vi "pendant_OC basic.vi"() -> ()   [LabVIEW 2014]
uses:
  <vilib>/Utility/miscctls.llb/LVBoundsTypeDef.ctl
  <vilib>/DAQmx/create/channels.llb/DAQmx Create Channel (AI-Voltage-Basic).vi
  <vilib>/DAQmx/configure/timing.llb/DAQmx Timing (Sample Clock).vi
  <vilib>/ethernetip/ethernetip.lvlib
panel:
  in  "Boolean 12":bool
  out "String 17":string="RECONNECT\nTRANSDUCER"
  out "Hz":dbl format="%05.1g"
  out "Trq":dbl format="%05.1g"
  in  "OK Button":bool
  out "Network Error":string="NETWORK\nERROR"
  out "DAQ READ ERROR":string
  out "HIMMELSTEIN READ ERROR":string
  out "DRIVE READ ERROR":string
  in  "Boolean 11":bool
  out "String 15":string="60HZ LOCK"
  in  "Boolean 7":bool=TRUE
  out "String 8":string="ADJ"
  in  "speed control":dbl(slide) max=100.0 step=0.1 scale=0.0..100.0 scale format="%05.1f"
  in  "Boolean 10":bool=TRUE
  out "String 9":string="ADJ"
  in  "trq control":dbl(slide) step=0.01 scale=0.0..100.0 scale format="%06.2g"
  in  "Boolean 9":bool
  in  "Boolean 5":bool
  out "String 14":string="RECONNECT\nTRANSDUCER"
  out "Numeric 10":dbl format="%_3g"
  out "2D Picture 7":picture
  out "String 13":string="PROBE\nERROR"
  out "String 12":string="TRANSDUCER\nERROR"
  out "String 10":string="ALARM"
  in  "Boolean 6":bool
  out "String 7":string="FAULT"
  out "Numeric 9":dbl format="%4_4g"
  out "2D Picture 6":picture
  in  "REV RUN":bool
  out "String 5":string="REV RUN"
  in  "FWD RUN":bool
  out "String 3":string="FWD RUN"
  in  "Boolean 3":bool
  out "String 4":string="STOP"
  out "Numeric 8":dbl format="%4_4g"
  out "2D Picture 5":picture
  out "Numeric 7":dbl format="%4_4g"
  out "2D Picture 4":picture
  out "Amps":dbl format="%05.1f"
  out "HP":dbl format="%05.1f"
  out "LB-FT":dbl format="%06.1f"
  out "RPM":dbl format="%06.1f"
  out "% Torque":dbl format="%05.1g"
  out "Hz":dbl format="%05.1g"
  in  "Dyne in use:":string(combo)
  in  "stop":bool
  out "Load Drive:":string
  # "Load Speed Actual:"
  # "Load Torque % Actual:"
  # "Speed \nRef/Lim (Hz)"
  # "Torque \nRef/Lim (%)"
  # "Current\nOnly"
  # "Average of 3 current probes"
  # "Yaskawa America, Inc."
  # "TEST DRIVE REGEN:\nset > test drive speed"
  # "Pendant style load controller"
  # "2018"
  # "v0.1"
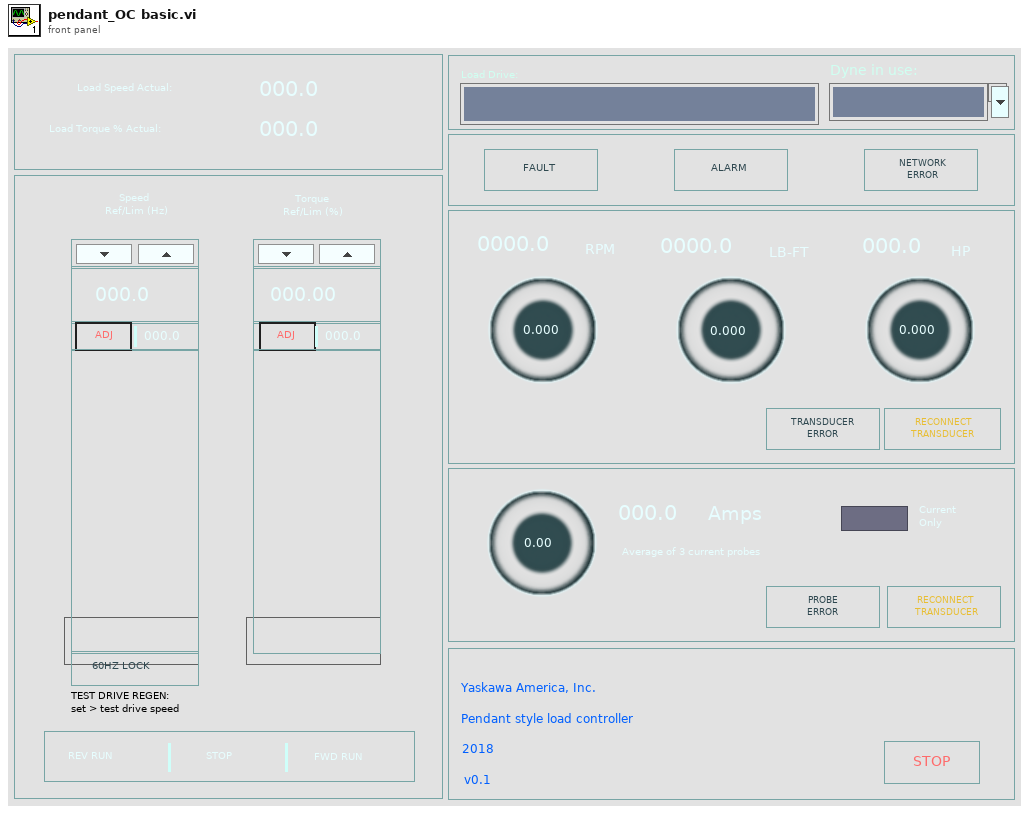
[diagram p1: front panel]
types:
  T1 = enum16{"[A1-02] Control Method Selection (general) [TEXT]", "[b1-01] Reference Source 1 (general) [TEXT]", "[b1-02] Run Source 1 (general) [TEXT]", "[b1-03] Stopping Method Selection (general) [TEXT]", "[C1-01] Acceleration Time 1 (general) [NUMERIC]", "[C1-02] Deceleration Time 1 (general) [NUMERIC]", "[C4-01] Torque Compensation Gain (general) [NUMERIC]", "[C6-01] Drive Duty Selection (general) [TEXT]", "[C6-02] Carrier Frequency Selection (general) [TEXT]", "[d1-01] Frequency Reference 1 (general) [NUMERIC]", "[H4-01] Multi-Function Analog Output Terminal FM Monitor Selection (general) [TEXT]", "[H4-02] Multi-Function Analog Output Terminal FM Gain (general) [NUMERIC]", "[H4-03] Multi-Function Analog Output Terminal FM Bias (general) [NUMERIC]", "[H4-04] Multi-Function Analog Output Terminal AM Monitor Selection (general) [TEXT]", "[H4-05] Multi-Function Analog Output Terminal AM Gain (general) [NUMERIC]", "[H4-06] Multi-Function Analog Output Terminal AM Bias (general) [NUMERIC]", "[L1-01] Motor Overload Protection Selection (general) [TEXT]", "[L3-01] Stall Prevention Selection during Acceleration (general) [TEXT]", "[L3-04] Stall Prevention Selection during Deceleration (general) [TEXT]", "[L3-05] Stall Prevention Selection during Run (general) [TEXT]", "[L8-14] Drive Overload (oL2) Protection Selection (general) [TEXT]", "[n1-01] Hunting Prevention Selection (general) [TEXT]", "[o2-04] Drive Model Selection (general) [TEXT]", "[C2-01] S-Curve Characteristic at Accel Start (S-Curve) [NUMERIC]", "[C2-02] S-Curve Characteristic at Accel End (S-Curve) [NUMERIC]", "[E1-03] V/f Pattern Selection (V/f Pattern) [TEXT]", "[E1-04] Maximum Output Frequency (V/f Pattern) [NUMERIC]", "[E1-05] Maximum Voltage (V/f Pattern) [NUMERIC]", "[E1-06] Base Frequency (V/f Pattern) [NUMERIC]", "[E1-07] Middle Output Frequency (V/f Pattern) [NUMERIC]", "[E1-08] Middle Output Frequency Voltage (V/f Pattern) [NUMERIC]", "[E1-09] Minimum Output Frequency (V/f Pattern) [NUMERIC]", "[E1-10] Minimum Output Frequency Voltage (V/f Pattern) [NUMERIC]", "[E2-01] Motor Rated Current (Motor Parameters) [NUMERIC]", "[E2-03] Motor No-Load Current (Motor Parameters) [NUMERIC]", "[E2-04] Number of Motor Poles (Motor Parameters) [NUMERIC]", "[E2-11] Motor Rated Power (Motor Parameters) [NUMERIC]", "[L1-13] Continuous Electrothermal Operation Selection (Memory Retention) [TEXT]", "[H1-01] Term S1 Func Sel (DI control) [TEXT]", "[H1-02] Term S2 Func Sel (DI control) [TEXT]", "[H1-03] Term S3 Func Sel (DI control) [TEXT]", "[H1-04] Term S4 Func Sel (DI control) [TEXT]", "[H1-05] Term S5 Func Sel (DI control) [TEXT]", "[H1-06] Term S6 Func Sel (DI control) [TEXT]", "[H1-07] Term S7 Func Sel (DI control) [TEXT]", "[H1-08] Term S8 Func Sel (DI control) [TEXT]", "[H3-01] Term A1 Level (AI control) [TEXT]", "[H3-02] Term A1 FuncSel (AI control) [TEXT]", "[H3-03] Term A1 Gain (AI control) [NUMERIC]", "[H3-04] Term A1 Bias (AI control) [NUMERIC]", "[H3-05] Term A3 Signal (AI control) [TEXT]", "[H3-06] Term A3 Sel (AI control) [TEXT]", "[H3-07] Term A3 Gain (AI control) [NUMERIC]", "[H3-08] Term A3 Bias (AI control) [NUMERIC]", "[H3-09] Term A2 Level (AI control) [TEXT]", "[H3-10] Term A2 FuncSel (AI control) [TEXT]", "[H3-11] Term A2 Gain (AI control) [NUMERIC]", "[H3-12] Term A2 Bias (AI control) [NUMERIC]"}
  T2 = enum16{"output frequency [U1-02]", "output current [U1-03]", "control method [U1-04]", "output voltage reference [U1-06]", "DC bus voltage [U1-07]", "output power [U1-08]"}
  T3 = typedef "LVBoundsTypeDef.ctl" = cluster{"Width":u32, "Height":u32}
  T4 = cluster{"Width":u32, "Width":u32, "Width":u32, "Height":u32}
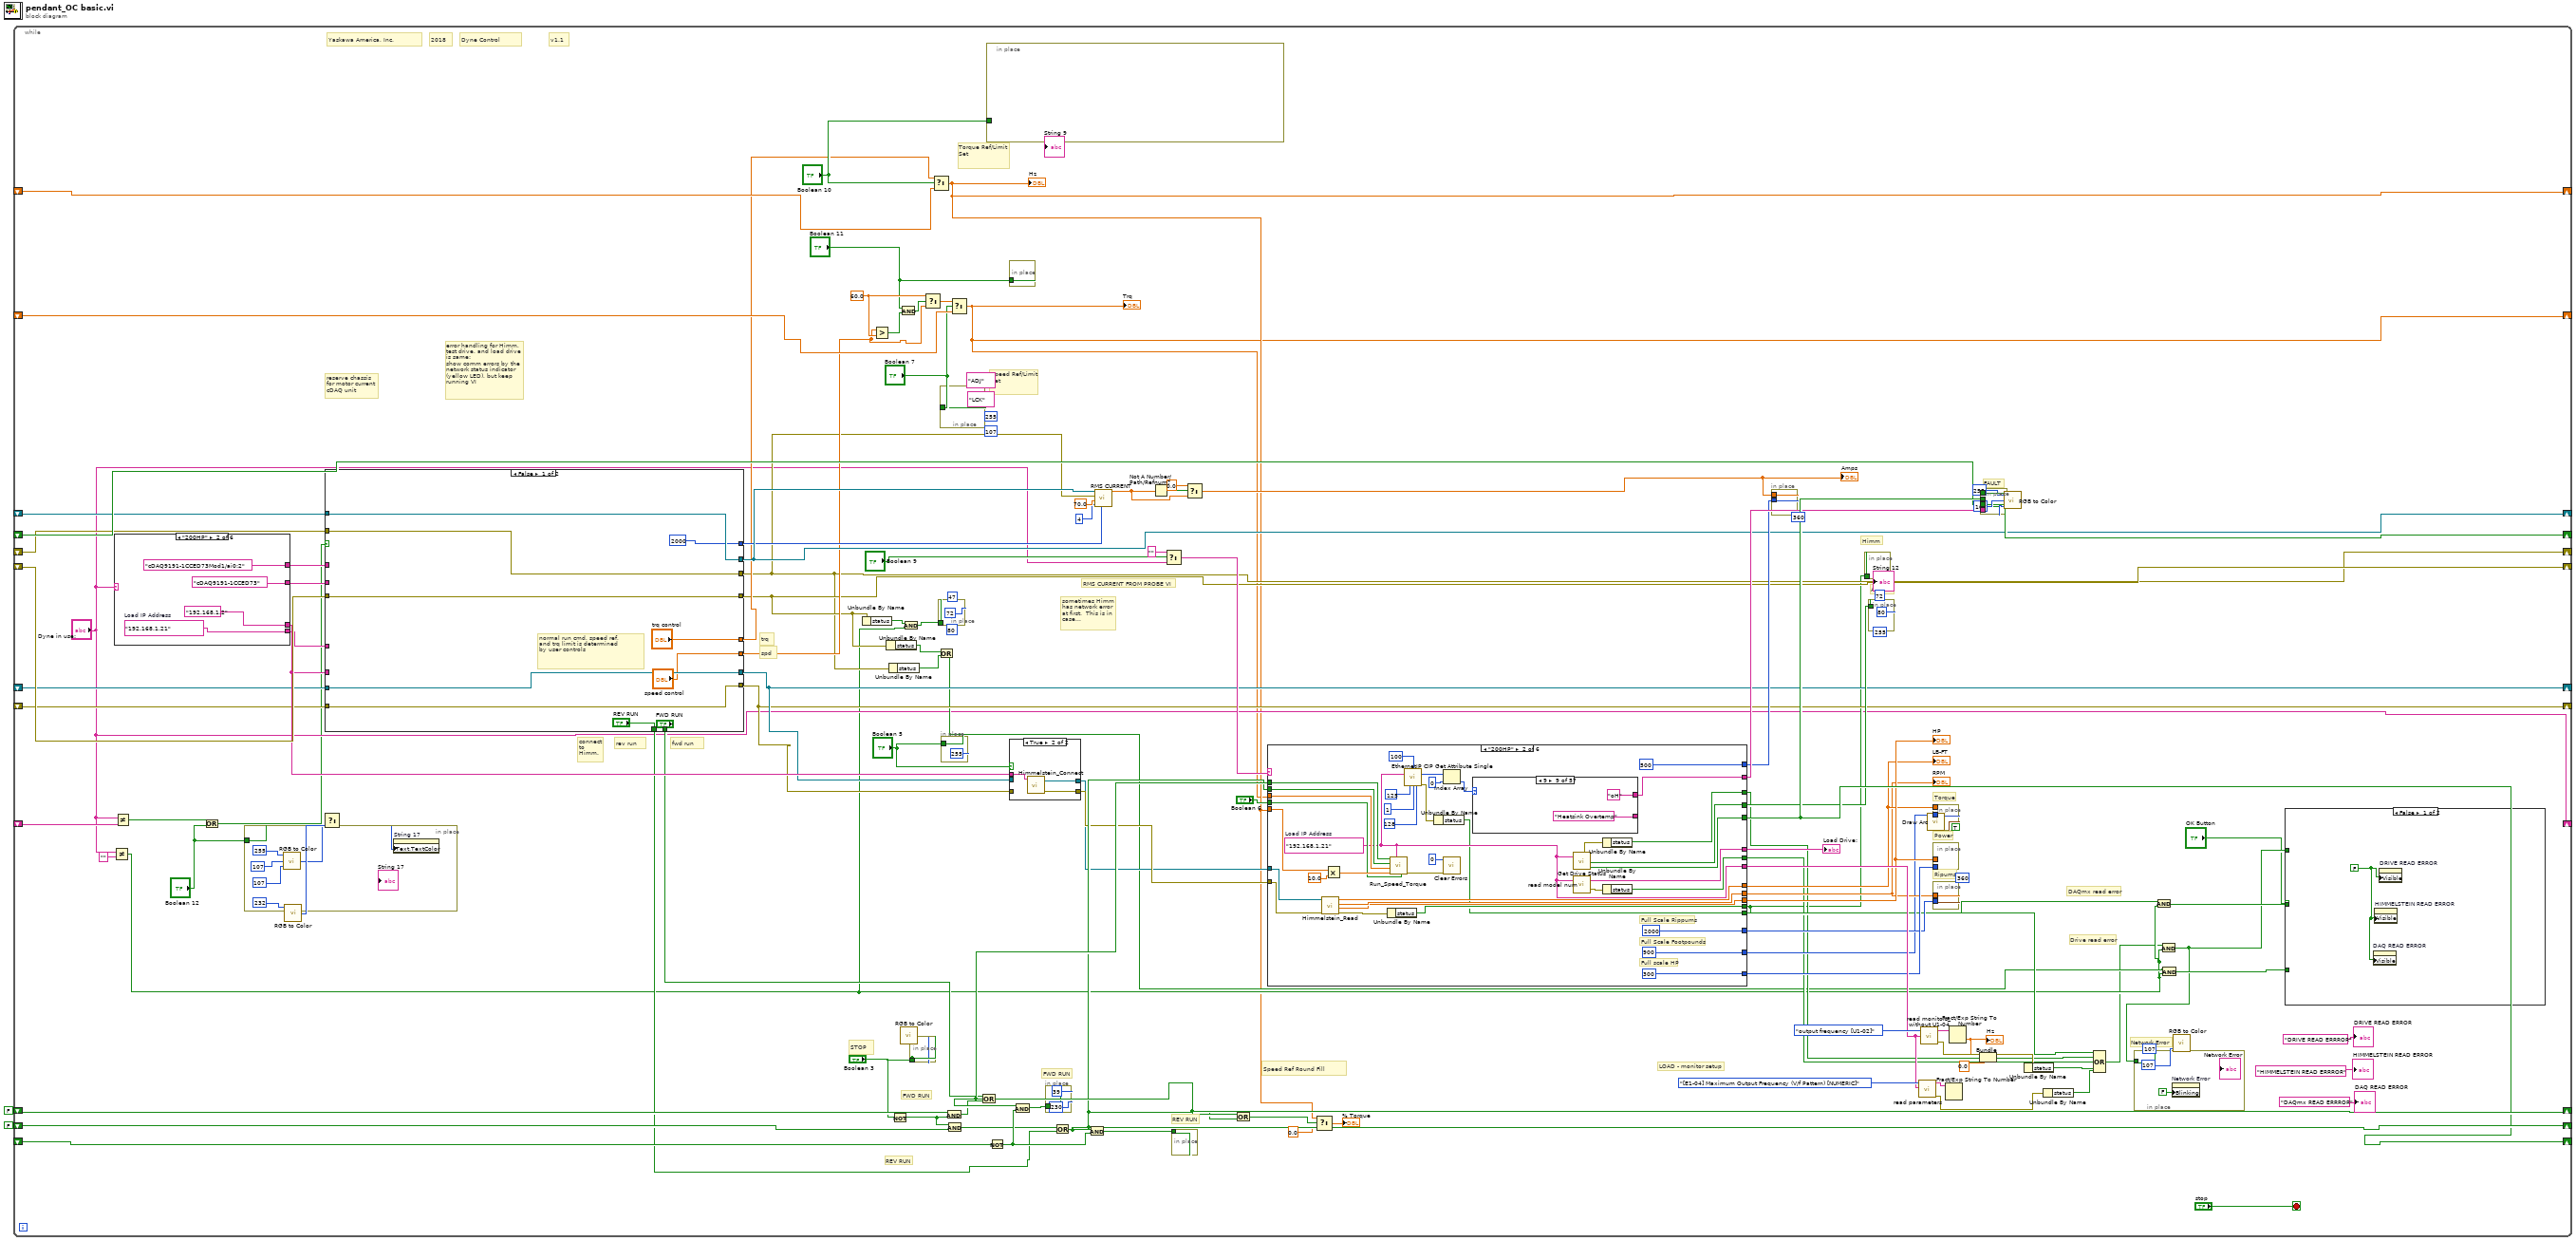
[diagram p0: block diagram]
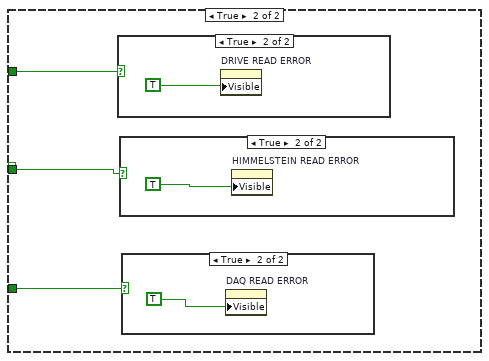
[diagram p2: hidden frame]
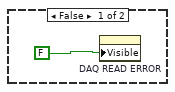
[diagram p3: hidden frame]
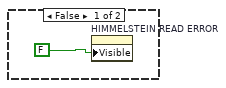
[diagram p4: hidden frame]
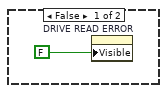
[diagram p5: hidden frame]
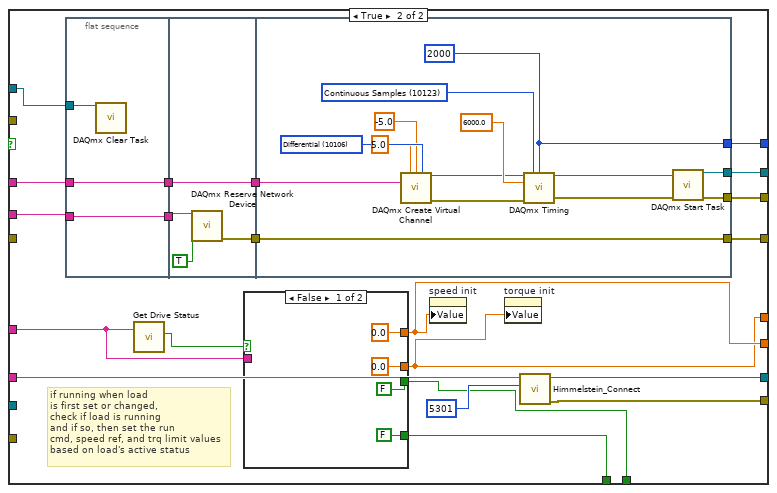
[diagram p6: hidden frame]
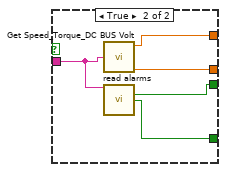
[diagram p7: hidden frame]
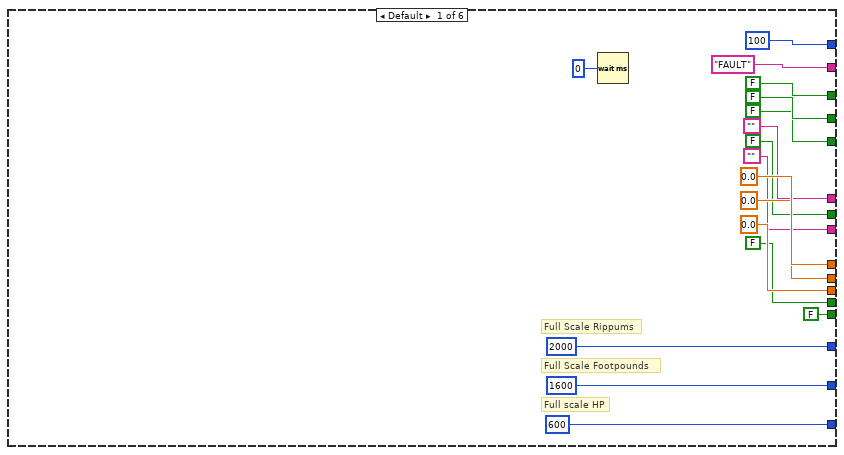
[diagram p9: hidden frame]
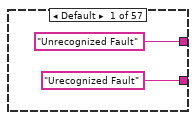
[diagram p10: hidden frame]
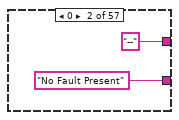
[diagram p11: hidden frame]
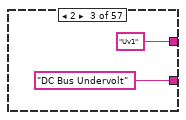
[diagram p12: hidden frame]
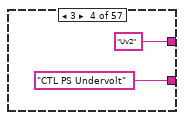
[diagram p13: hidden frame]
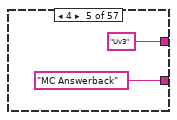
[diagram p14: hidden frame]
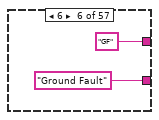
[diagram p15: hidden frame]
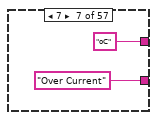
[diagram p16: hidden frame]
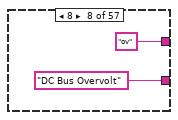
[diagram p17: hidden frame]
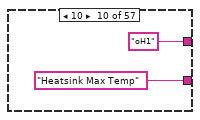
[diagram p18: hidden frame]
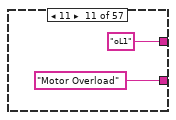
[diagram p19: hidden frame]
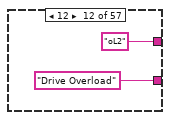
[diagram p20: hidden frame]
diagram:
  n1 = while {
    shift-right: [w107] -> _
    shift-left: FALSE -> [w104]
    shift-right: [w106] -> _
    shift-left: FALSE -> [w103]
    shift-right: [w105] -> _
    shift-left: _ -> [w102]
    shift-right: [w7] -> _
    shift-left: _ -> [w100]
    shift-right: [w6] -> _
    shift-left: _ -> [w101]
    shift-right: [w99] -> _
    shift-left: _ -> [w98]
    shift-right: ["Dyne in use:"] -> _
    shift-left: _ -> [w53]
    shift-right: [w25] -> _
    shift-left: _ -> [w50]
    shift-right: [w52] -> _
    shift-left: _ -> [w51]
    shift-right: [w26] -> _
    shift-left: _ -> [w49]
    shift-right: [w46] -> _
    shift-left: _ -> [w44]
    shift-right: [w45] -> _
    shift-left: _ -> [w43]
    stop <- "stop" stop-if-true
    w73 = 60.0 ("t")
    # "DAQmx read error"
    # "Drive read error"
    # "rev run"
    # "fwd run"
    # "spd"
    # "trq"
    # "REV RUN"
    # "FWD RUN"
    # "Network Error"
    # "ALARM"
    # "REV RUN"
    # "STOP"
    # "sometimes Himm\nhas network error \nat first.  This is in\ncase..."
    # "Speed Ref Round Fill"
    # "Speed Ref/Limit Set"
    # "Torque Ref/Limit Set"
    # "FAULT"
    # "FWD RUN"
    # "LOAD - monitor setup"
    # "Himm"
    # "RMS CURRENT FROM PROBE VI"
    # "Torque"
    # "Power"
    # "Ripums"
    # "reserve chassis \nfor motor current\ncDAQ unit"
    # "error handling for Himm,\ntest drive, and load drive\nis same:\nshow comm errors by the \nnetwork status indicator \n(yellow LED), but keep\nrunning VI"
    # "connect\nto \nHimm."
    # "Dyne Control"
    # "v1.1"
    # "2018"
    # "Yaskawa America, Inc."
    n2 = Not Equal?(x="Dyne in use:", y="") -> (x != y?=w11:bool)
    n3 = case shown="\"200HP\"" "Dyne in use:" {
      tunnel: [tag "" ("device in") tag "cDAQ9191-1CCED73" ("device in") tag "" ("device in") tag "cDAQ9191-1CCED79" ("device in") tag "cDAQ9191-1CCED73" ("device in") tag "cDAQ9191-1CCED73" ("device in")] -> w109
      tunnel: ["" "192.168.1.2" "" "192.168.1.3" "192.168.1.5" "192.168.1.4"] -> w47
      tunnel: [tag "" ("physical channels") tag "cDAQ9191-1CCED73Mod1/ai0:2" ("physical channels") tag "" ("physical channels") tag "cDAQ9191-1CCED79Mod1/ai0:2" ("physical channels") tag "cDAQ9191-1CCED73Mod1/ai0:2" ("physical channels") tag "cDAQ9191-1CCED73Mod1/ai0:2" ("physical channels")] -> w108
      tunnel: [w1160 w1164 w1168 w1172 w1176 w1180] -> w36
      frame Default {
        w1160 = ""  # Load IP Address
      }
      frame "200HP" {
        w1164 = "192.168.1.21"  # Load IP Address
      }
      frame "Portable Stand" {
        w1168 = "192.168.1.20"  # Load IP Address
      }
      frame "500HP" {
        w1172 = "192.168.1.22"  # Load IP Address
      }
      frame "1200HP" {
        w1176 = "192.168.1.23"  # Load IP Address
      }
      frame "600HP" {
        w1180 = "192.168.1.23"  # Load IP Address
      }
    }
    n4 = Not Equal?(x="Dyne in use:", y=w53) -> (x != y?=w5:bool)
    n5 = Or(x=w5, y="Boolean 12") -> (x .or. y?=w4:bool)
    n6 = in-place {
      in-place-border: "Boolean 12" -> [w113]
      # "reconnect"
      n7 = call <vilib>:"RGB to Color.vi"("B"=u8 107 ("R"), "G"=u8 107 ("R"), "R"=u8 255) -> ("Color"=w111:u32)
      n8 = call <vilib>:"RGB to Color.vi"("B"=u8 51 ("R"), "G"=u8 190 ("R"), "R"=u8 232) -> ("Color"=w112:u32)
      n9 = Select(t=w111, s=w113, f=w112) -> (s? t:f=w110:u32)
      n10 = property on="String 17" class="Str"("Text.TextColor"=w110) -> ()  [unwired: 2 in, 2 out]
    }
    n11 = case shown="False" w4 {
      tunnel: w109 -> [_ w158]
      tunnel: [w137 w157] -> w26
      tunnel: w108 -> [_ w156]
      tunnel: [w139 w155] -> w52
      tunnel: [w138 w154] -> w25
      tunnel: w51 -> [w139 w146]
      tunnel: w50 -> [w138 _]
      tunnel: w49 -> [w137 _]
      tunnel: [w136 w153] -> w46
      tunnel: [w135 w152] -> w45
      tunnel: w47 -> [_ w151]
      tunnel: w44 -> [w136 _]
      tunnel: w43 -> [w135 _]
      tunnel: [2000 ("samples per channel") w149] -> w37
      tunnel: w36 -> [_ w144]
      tunnel: ["trq control" w142] -> w35
      tunnel: ["speed control" w143] -> w34
      tunnel: ["FWD RUN" w140] -> w33
      tunnel: ["REV RUN" w141] -> w32
      frame False {
        # "normal run cmd, speed ref,\nand trq limit is determined\nby user controls"
      }
      frame True {
        # "if running when load \nis first set or changed, \ncheck if load is running\nand if so, then set the run\ncmd, speed ref, and trq limit values\nbased on load's active status"
        n12 = flat-sequence {
          tunnel: w156 -> [w171]
          tunnel: w158 -> [w172]
          tunnel: [w172] -> w148
          tunnel: [w171] -> w147
          tunnel: w146 -> [w170]
          tunnel: [w175] -> w160
          tunnel: [w174] -> w159
          tunnel: w148 -> [w176]
          tunnel: w147 -> [w174]
          tunnel: w160 -> [w190]
          tunnel: [w190] -> w157
          tunnel: w159 -> [w182]
          tunnel: [w181] -> w155
          tunnel: [w180] -> w154
          tunnel: [w177] -> w149
          frame #0 {
            n13 = call <vilib>:"DAQmx Clear Task.vi"("task in"=w170) -> ()  [unwired: 14 in, 1 out]
          }
          frame #1 {
            n14 = call <vilib>:"DAQmx Reserve Network Device.vi"("device in"=w176, "override reservation?"=TRUE) -> ("error out"=w175:errorcluster)  [unwired: 12 in, 1 out]
          }
          frame #2 {
            w189 = 10106 items=["Default"=-1, "RSE"=10083, "NRSE"=10078, "Differential"=10106, "Pseudodifferential"=12529] ("input terminal configuration")
            w185 = 10123 items=["Finite Samples"=10178, "Continuous Samples"=10123, "Hardware Timed Single Point"=12522] ("sample mode")
            w177 = 2000 ("samples per channel")
            n15 = call-poly <vilib>:"DAQmx Create Virtual Channel.vi"("maximum value"=5.0, "minimum value"=-5.0, "input terminal configuration"=w189, "physical channels"=w182) -> ("task out"=w183:refnum<k21>, "error out"=w184:errorcluster)  [unwired: 10 in]
            n16 = call-poly <vilib>:"DAQmx Timing.vi"("task/channels in"=w183, "sample mode"=w185, "samples per channel"=w177, "rate"=6000.0, "error in"=w184) -> ("task out"=w179:refnum<k21>, "error out"=w178:errorcluster)  [unwired: 9 in]
            n17 = call <vilib>:"DAQmx Start Task.vi"("task/channels in"=w179, "error in"=w178) -> ("task out"=w181:refnum<k21>, "error out"=w180:errorcluster)  [unwired: 12 in]
          }
        }
        n18 = call "Get Drive Status.vi"("Network Path"=w144) -> ("Running"=w145:bool)  [unwired: 1 in, 4 out]
        n19 = case shown="False" w145 {
          tunnel: w144 -> [_ w167]
          tunnel: [0.0 ("Actual Torque (%)") w169] -> w142
          tunnel: [0.0 ("Output Freq") w168] -> w143
          tunnel: [FALSE ("FWD RUN") w166] -> w140
          tunnel: [FALSE ("REV RUN") w165] -> w141
          frame False {
          }
          frame True {
            n20 = call "Get Speed_Torque_DC BUS Volt.vi"("Network Path"=w167) -> ("Output Freq"=w168:dbl, "Actual Torque (%)"=w169:dbl)  [unwired: 1 in, 4 out]
            n21 = call "read alarms.vi"("A1000 IP address"=w167) -> ("FWD RUN"=w166:bool, "REV RUN"=w165:bool)  [unwired: 7 in, 6 out]
          }
        }
        n22 = property on="speed init" class="Slide (strict)"("Value"=w143) -> ()  [unwired: 2 in, 2 out]
        n23 = property on="torque init" class="Slide (strict)"("Value"=w142) -> ()  [unwired: 2 in, 2 out]
        n24 = call "Himmelstein_Connect.vi"("remote port"=u16 5301, "IP Address"=w151) -> ("error out"=w152:errorcluster, "connection ID"=w153:refnum<k5>)  [unwired: 8 in]
      }
    }
    n25 = Unbundle By Name(w26) -> ("status"=w13:bool)
    n26 = Greater?(x=w34, y=w73) -> (0:w72:bool)
    n27 = Unbundle By Name(w26) -> ("status"=w24:bool)
    n28 = Unbundle By Name(w25) -> ("status"=w23:bool)
    n29 = Not(x="Boolean 3") -> (.not. x?=w58:bool)
    n30 = And(x="Boolean 11", y=w72) -> (x .and. y?=w71:bool)
    n31 = And(x=w13, y=w11) -> (x .and. y?=w12:bool)
    n32 = in-place {
      in-place-border: "Boolean 3" -> [w371]
      n33 = call <vilib>:"RGB to Color.vi"("B"=u8 107 ("R"), "G"=u8 107 ("R"), "R"=u8 255) -> ("Color"=w359:u32)
      n34 = call <vilib>:"RGB to Color.vi"("B"=u8 255 ("R"), "G"=u8 254 ("R"), "R"=u8 231) -> ("Color"=w360:u32)
      n35 = Select(t=w359, s=w371, f=w360) -> (s? t:f=w363:u32)
      n36 = Select(t="STOP" ("Text.Text"), s=w371, f="STOP" ("Text.Text")) -> (s? t:f=w362:string)
      n37 = property on="String 4" class="Str"("Text.TextColor"=w363) -> ()  [unwired: 2 in, 2 out]
      n38 = property on="String 4" class="Str"("Text.Text"=w362) -> ()  [unwired: 2 in, 2 out]
    }
    n39 = Select(t=w73, s=w71, f=w34) -> (s? t:f=w70:dbl)
    n40 = Select(t=w35, s="Boolean 10", f=w100) -> (s? t:f=w7:dbl)
    "Hz" <- w7
    n41 = Or(x=w24, y=w23) -> (x .or. y?=w19:bool)
    n42 = in-place {
      in-place-border: w12 -> [w202]
      # "fwd run"
      n43 = call <vilib>:"RGB to Color.vi"("B"=u8 80 ("R"), "G"=u8 72 ("R"), "R"=u8 47) -> ("Color"=w206:u32)
      n44 = call <vilib>:"RGB to Color.vi"("B"=u8 107 ("R"), "G"=u8 107 ("R"), "R"=u8 255) -> ("Color"=w210:u32)
      n45 = Select(t=w210, s=w202, f=w206) -> (s? t:f=w201:u32)
      n46 = property on="String 13" class="Str"("Text.TextColor"=w201) -> ()  [unwired: 2 in, 2 out]
    }
    n47 = in-place {
      in-place-border: "Boolean 7" -> [w324]
      n48 = Select(t="ADJ" ("Text.Text"), s=w324, f="LCK" ("Text.Text")) -> (s? t:f=w312:string)
      n49 = call <vilib>:"RGB to Color.vi"("B"=u8 51 ("R"), "G"=u8 190 ("R"), "R"=u8 232) -> ("Color"=w314:u32)
      n50 = call <vilib>:"RGB to Color.vi"("B"=u8 107 ("R"), "G"=u8 107 ("R"), "R"=u8 255) -> ("Color"=w315:u32)
      n51 = Select(t=w314, s=w324, f=w315) -> (s? t:f=w313:u32)
      n52 = property on="String 8" class="Str"("Text.Text"=w312) -> ()  [unwired: 2 in, 2 out]
      n53 = property on="String 8" class="Str"("Text.TextColor"=w313) -> ()  [unwired: 2 in, 2 out]
    }
    n54 = in-place {
      in-place-border: "Boolean 5" -> [w375]
      # "reconnect"
      n55 = call <vilib>:"RGB to Color.vi"("B"=u8 107 ("R"), "G"=u8 107 ("R"), "R"=u8 255) -> ("Color"=w372:u32)
      n56 = call <vilib>:"RGB to Color.vi"("B"=u8 51 ("R"), "G"=u8 190 ("R"), "R"=u8 232) -> ("Color"=w373:u32)
      n57 = Select(t=w372, s=w375, f=w373) -> (s? t:f=w374:u32)
      n58 = property on="String 14" class="Str"("Text.TextColor"=w374) -> ()  [unwired: 2 in, 2 out]
    }
    n59 = And(x=w104, y=w58) -> (x .and. y?=w97:bool)
    n60 = And(x=w58, y=w103) -> (x .and. y?=w57:bool)
    n61 = Select(t=w70, s="Boolean 7", f=w101) -> (s? t:f=w6:dbl)
    "Trq" <- w6
    n62 = Or(x=w33, y=w97) -> (x .or. y?=w107:bool)
    n63 = in-place {
      in-place-border: "Boolean 10" -> [w311]
      n64 = Select(t="ADJ" ("Text.Text"), s=w311, f="LCK" ("Text.Text")) -> (s? t:f=w299:string)
      n65 = property on="String 9" class="Str"("Text.Text"=w299) -> ()  [unwired: 2 in, 2 out]
      n66 = call <vilib>:"RGB to Color.vi"("B"=u8 51 ("R"), "G"=u8 190 ("R"), "R"=u8 232) -> ("Color"=w301:u32)
      n67 = call <vilib>:"RGB to Color.vi"("B"=u8 107 ("R"), "G"=u8 107 ("R"), "R"=u8 255) -> ("Color"=w302:u32)
      n68 = Select(t=w301, s=w311, f=w302) -> (s? t:f=w300:u32)
      n69 = property on="String 9" class="Str"("Text.TextColor"=w300) -> ()  [unwired: 2 in, 2 out]
    }
    n70 = Not(x=w102) -> (.not. x?=w81:bool)
    n71 = in-place {
      in-place-border: "Boolean 11" -> [w200]
      n72 = call <vilib>:"RGB to Color.vi"("B"=u8 255 ("R"), "G"=u8 254 ("R"), "R"=u8 231) -> ("Color"=w193:u32)
      n73 = call <vilib>:"RGB to Color.vi"("B"=u8 80 ("R"), "G"=u8 72 ("R"), "R"=u8 47) -> ("Color"=w192:u32)
      n74 = Select(t=w193, s=w200, f=w192) -> (s? t:f=w191:u32)
      n75 = property on="String 15" class="Str"("Text.TextColor"=w191) -> ()  [unwired: 2 in, 2 out]
    }
    n76 = case shown="True" "Boolean 5" {
      tunnel: [w383 w385] -> w87
      tunnel: w45 -> [w383 _]
      tunnel: w46 -> [w382 _]
      tunnel: [w382 w386] -> w86
      tunnel: w47 -> [_ w384]
      frame False {
      }
      frame True {
        n77 = call "Himmelstein_Connect.vi"("IP Address"=w384) -> ("error out"=w385:errorcluster, "connection ID"=w386:refnum<k5>)  [unwired: 9 in]
      }
    }
    n78 = And(x=w107, y=w81) -> (x .and. y?=w75:bool)
    n79 = in-place {
      in-place-border: w75 -> [w339]
      n80 = call <vilib>:"RGB to Color.vi"("B"=u8 255 ("R"), "G"=u8 254 ("R"), "R"=u8 231) -> ("Color"=w343:u32)
      n81 = call <vilib>:"RGB to Color.vi"("B"=u8 118 ("R"), "G"=u8 230 ("R"), "R"=u8 39) -> ("Color"=w347:u32)
      n82 = Select(t=w347, s=w339, f=w343) -> (s? t:f=w348:u32)
      n83 = property on="String 3" class="Str"("Text.TextColor"=w348) -> ()  [unwired: 2 in, 2 out]
    }
    n84 = Or(x=w57, y=w32) -> (x .or. y?=w106:bool)
    n85 = And(x=w106, y=w81) -> (x .and. y?=w74:bool)
    n86 = call "RMS CURRENT.vi"("number of samples per channel"=w37, "order"=4, "cutoff frequency"=70.0, "error in (no error)"=w25, "task out"=w52) -> ("RMS Value Average"=w61:dbl)  [unwired: 2 in, 4 out]
    n87 = Not A Number/Path/Refnum?(number/path/refnum=w61) -> (NaN/Path/Refnum?=w62:bool)
    n88 = Select(t="", s="Boolean 9", f="Dyne in use:") -> (s? t:f=w56:string)
    n89 = in-place {
      in-place-border: w74 -> [w358]
      n90 = call <vilib>:"RGB to Color.vi"("B"=u8 255 ("R"), "G"=u8 254 ("R"), "R"=u8 231) -> ("Color"=w349:u32)
      n91 = call <vilib>:"RGB to Color.vi"("B"=u8 118 ("R"), "G"=u8 230 ("R"), "R"=u8 39) -> ("Color"=w350:u32)
      n92 = Select(t=w350, s=w358, f=w349) -> (s? t:f=w357:u32)
      n93 = property on="String 5" class="Str"("Text.TextColor"=w357) -> ()  [unwired: 2 in, 2 out]
    }
    n94 = Select(t=0.0, s=w62, f=w61) -> (s? t:f=w59:dbl)
    "Amps" <- w59
    n95 = Or(x=w107, y=w106) -> (x .or. y?=w79:bool)
    n96 = case shown="\"200HP\"" w56 {
      tunnel: w6 -> [_ w431 w582 w732 w888 w1039]
      tunnel: w107 -> [_ w429 w580 w731 w882 w1033]
      tunnel: [0.0 ("Torque") w425 w574 w725 w876 w1027] -> w66
      tunnel: [0.0 ("Speed") w424 w576 w727 w877 w1028] -> w65
      tunnel: [0.0 ("Power") w423 w575 w726 w878 w1029] -> w77
      tunnel: [FALSE ("status") w435 w586 w743 w887 w1038] -> w17
      tunnel: w7 -> [_ w432 w583 w734 w883 w1034]
      tunnel: w86 -> [_ w428 w579 w730 w881 w1032]
      tunnel: w87 -> [_ w427 w578 w729 w880 w1031]
      tunnel: "Boolean 6" -> [_ w433 w585 w735 w886 w1037]
      tunnel: w106 -> [_ w430 w581 w733 w884 w1035]
      tunnel: ["" w434 w584 w742 w885 w1036] -> w92
      tunnel: ["" w412 w557 w714 w859 w1010] -> w90
      tunnel: [FALSE ("Alarm") w422 w572 w723 w874 w1025] -> w76
      tunnel: [FALSE ("Fault") w421 w573 w724 w875 w1026] -> w105
      tunnel: [FALSE ("status") w420 w571 w722 w873 w1024] -> w27
      tunnel: [FALSE ("status") w419 w570 w721 w872 w1023] -> w28
      tunnel: ["FAULT" w411 w556 w713 w858 w1009] -> w69
      tunnel: [u16 2000 ("y") u16 2000 ("y") u16 2000 ("y") u16 2000 ("y") u16 2000 ("y") u16 2000 ("y")] -> w64
      tunnel: [1600 900 100 1600 3300 1600] -> w63
      tunnel: [600 300 20 600 1250 600] -> w68
      tunnel: [u16 100 ("y") 500 50 600 1500 1000] -> w67
      tunnel: [FALSE ("status") w405 FALSE ("status") w707 FALSE ("status") FALSE ("status")] -> w29
      frame Default {
        # "Full scale HP"
        # "Full Scale Footpounds"
        # "Full Scale Rippums"
        n97 = Wait (ms)(milliseconds to wait=u32 0) -> ()  [unwired: 1 out]
      }
      frame "200HP" {
        w412 = "192.168.1.21"  # Load IP Address
        # "Full scale HP"
        # "Full Scale Footpounds"
        # "Full Scale Rippums"
        n98 = call "Himmelstein_Read.vi"("connection ID"=w428, "error in (no error)"=w427) -> ("Torque"=w425:dbl, "Speed"=w424:dbl, "Power"=w423:dbl, "error out"=w426:errorcluster)  [unwired: 2 in, 1 out]
        n99 = Multiply(x=w432, y=10.0) -> (x*y=w436:dbl)
        n100 = Unbundle By Name(w426) -> ("status"=w435:bool)
        n101 = call "Run_Speed_Torque.vi"("Fault reset"=w433, "Network Path"=w412, "Torque Limit"=w436, "Speed Reference"=w431, "RUN REV."=w430, "RUN FOR."=w429) -> ("error out"=w438:errorcluster)  [unwired: 4 in, 1 out]
        n102 = call <vilib>:"EthernetIP CIP Get Attribute Single.vi"("Timeout (ms)"=100, "Network Path"=w412, "Class"=125, "Instance"=u32 1, "Attribute"=128) -> ("Data"=w415:u8[], "error out"=w406:errorcluster)  [unwired: 8 in, 1 out]
        n103 = Unbundle By Name(w406) -> ("status"=w405:bool)
        n104 = Index Array(array=w415, index=0) -> (element=w413:u8)
        n105 = call <vilib>:"Clear Errors.vi"("error in (no error)"=w438, "specific error code to clear (0: all)"=0) -> ()  [unwired: 4 in, 2 out]
        n106 = case shown="9" w413 {
          tunnel: ["Unrecognized Fault" "--" "Uv1" "Uv2" "Uv3" "GF" "oC" "ov" "oH" "oH1" "oL1" "oL2" "oL3" "oL4" "rr" "rH" "EF3" "EF4" "EF5" "EF6" "EF7" "EF8" "oS" "dEv" "PGo" "PF" "LF" "oH3" "oPr" "Err" "oH4" "CE" "bUS" "CF" "EF0" "FbL" "UL3" "UL4" "oL7" "dv1" "dv2" "dv3" "dv4" "LF2" "STo" "PGoH" "SEr" "FbH" "EF1" "EF2" "oL5" "UL5" "CoF" "dwFL" "voF" "rF" "boL"] -> w411
          tunnel: ["Urecognized Fault" "No Fault Present" "DC Bus Undervolt" "CTL PS Undervolt" "MC Answerback" "Ground Fault" "Over Current" "DC Bus Overvolt" "Heatsink Overtemp" "Heatsink Max Temp" "Motor Overload" "Drive Overload" "Overtorque Det 1" "Overtorque Det 2" "DynBrk Transistor" "DynBrk Resistor" "External Fault 3" "External Fault 4" "External Fault 5" "External Fault 6" "External Fault 7" "External Fault 8" "Overspeed Det" "Speed Deviation" "PG Open" "Input Phase Loss" "Output Phase Loss" "Motor Overheat 1 (PTC Input)" "Operator Disconnected" "EEPROM R/W Error" "Motor OverHeat 2 (PTC Input)" "MEMOBUS/Modbus Com Fault" "EtherNet/IP Communication Error" "Out of Control" "External Fault 0" "PID Feedback Loss" "Undertorque Detection 1" "Undertorque Detection 2" "High Slip Braking oL" "Z Pulse Fault Detection" "Z pulse Noise Fault Detection" "Inversion Detection" "Inversion Prevention Detection" "Current Imbalance" "Pull-Out Detection" "PG Hardware Fault" "Too Many Speed Search Restarts" "Excessive PID Feedback" "External Fault (input terminal S1)" "External Fault (input terminal S2)" "Mechanical WeakeningDetection 1" "Mechanical Weakening Detection 2" "Current Offset Fault" "DriveWorksEZ Fault" "Output Voltage Detection Fault" "Braking Resistor Fault" "Braking Transistor Overload Fault"] -> _
          frame Default {
          }
          frame 0 {
          }
          frame 2 {
          }
          frame 3 {
          }
          frame 4 {
          }
          frame 6 {
          }
          frame 7 {
          }
          frame 8 {
          }
          frame 9 {
          }
          frame 10 {
          }
          frame 11 {
          }
          frame 12 {
          }
          frame 13 {
          }
          frame 14 {
          }
          frame 15 {
          }
          frame 16 {
          }
          frame 17 {
          }
          frame 18 {
          }
          frame 19 {
          }
          frame 20 {
          }
          frame 21 {
          }
          frame 22 {
          }
          frame 24 {
          }
          frame 25 {
          }
          frame 26 {
          }
          frame 27 {
          }
          frame 28 {
          }
          frame 29 {
          }
          frame 30 {
          }
          frame 31 {
          }
          frame 32 {
          }
          frame 33 {
          }
          frame 34 {
          }
          frame 37 {
          }
          frame 39 {
          }
          frame 40 {
          }
          frame 41 {
          }
          frame 42 {
          }
          frame 43 {
          }
          frame 50 {
          }
          frame 51 {
          }
          frame 52 {
          }
          frame 53 {
          }
          frame 54 {
          }
          frame 55 {
          }
          frame 56 {
          }
          frame 59 {
          }
          frame 65 {
          }
          frame 66 {
          }
          frame 67 {
          }
          frame 68 {
          }
          frame 69 {
          }
          frame 70 {
          }
          frame 73 {
          }
          frame 77 {
          }
          frame 78 {
          }
          frame 79 {
          }
        }
        n107 = call "Get Drive Status.vi"("Network Path"=w412) -> ("Fault"=w421:bool, "Alarm"=w422:bool, "error out"=w440:errorcluster)  [unwired: 1 in, 2 out]
        n108 = call "read model num.vi"("A1000 IP address"=w412) -> ("error out"=w441:errorcluster, "model string"=w434:string)  [unwired: 1 in]
        n109 = Unbundle By Name(w440) -> ("status"=w419:bool)
        n110 = Unbundle By Name(w441) -> ("status"=w420:bool)
      }
      frame "Portable Stand" {
        w557 = "192.168.1.20"  # Load IP Address
        # "Full scale HP"
        # "Full Scale Footpounds"
        # "Full Scale Rippums"
        n111 = call <vilib>:"EthernetIP CIP Get Attribute Single.vi"("Network Path"=w557, "Class"=125, "Instance"=u32 1, "Attribute"=128) -> ("Data"=w561:u8[], "error out"=w558:errorcluster)  [unwired: 9 in, 1 out]
        n112 = Unbundle By Name(w558) -> ()  [unwired: 1 out]
        n113 = call "Himmelstein_Read.vi"("connection ID"=w579, "error in (no error)"=w578) -> ("Torque"=w574:dbl, "Speed"=w576:dbl, "Power"=w575:dbl, "error out"=w577:errorcluster)  [unwired: 2 in, 1 out]
        n114 = Index Array(array=w561, index=0) -> (element=w559:u8)
        n115 = Multiply(x=w583, y=10.0) -> (x*y=w587:dbl)
        n116 = case shown="56" w559 {
          tunnel: ["Unrecognized Fault" "--" "Uv1" "Uv2" "Uv3" "GF" "oC" "ov" "oH" "oH1" "oL1" "oL2" "oL3" "oL4" "rr" "rH" "EF3" "EF4" "EF5" "EF6" "EF7" "EF8" "oS" "dEv" "PGo" "PF" "LF" "oH3" "oPr" "Err" "oH4" "CE" "bUS" "CF" "EF0" "FbL" "UL3" "UL4" "oL7" "dv1" "dv2" "dv3" "dv4" "LF2" "STo" "PGoH" "SEr" "FbH" "EF1" "EF2" "oL5" "UL5" "CoF" "dwFL" "voF" "rF" "boL"] -> w556
          tunnel: ["Urecognized Fault" "No Fault Present" "DC Bus Undervolt" "CTL PS Undervolt" "MC Answerback" "Ground Fault" "Over Current" "DC Bus Overvolt" "Heatsink Overtemp" "Heatsink Max Temp" "Motor Overload" "Drive Overload" "Overtorque Det 1" "Overtorque Det 2" "DynBrk Transistor" "DynBrk Resistor" "External Fault 3" "External Fault 4" "External Fault 5" "External Fault 6" "External Fault 7" "External Fault 8" "Overspeed Det" "Speed Deviation" "PG Open" "Input Phase Loss" "Output Phase Loss" "Motor Overheat 1 (PTC Input)" "Operator Disconnected" "EEPROM R/W Error" "Motor OverHeat 2 (PTC Input)" "MEMOBUS/Modbus Com Fault" "EtherNet/IP Communication Error" "Out of Control" "External Fault 0" "PID Feedback Loss" "Undertorque Detection 1" "Undertorque Detection 2" "High Slip Braking oL" "Z Pulse Fault Detection" "Z pulse Noise Fault Detection" "Inversion Detection" "Inversion Prevention Detection" "Current Imbalance" "Pull-Out Detection" "PG Hardware Fault" "Too Many Speed Search Restarts" "Excessive PID Feedback" "External Fault (input terminal S1)" "External Fault (input terminal S2)" "Mechanical WeakeningDetection 1" "Mechanical Weakening Detection 2" "Current Offset Fault" "DriveWorksEZ Fault" "Output Voltage Detection Fault" "Braking Resistor Fault" "Braking Transistor Overload Fault"] -> _
          frame Default {
          }
          frame 0 {
          }
          frame 2 {
          }
          frame 3 {
          }
          frame 4 {
          }
          frame 6 {
          }
          frame 7 {
          }
          frame 8 {
          }
          frame 9 {
          }
          frame 10 {
          }
          frame 11 {
          }
          frame 12 {
          }
          frame 13 {
          }
          frame 14 {
          }
          frame 15 {
          }
          frame 16 {
          }
          frame 17 {
          }
          frame 18 {
          }
          frame 19 {
          }
          frame 20 {
          }
          frame 21 {
          }
          frame 22 {
          }
          frame 24 {
          }
          frame 25 {
          }
          frame 26 {
          }
          frame 27 {
          }
          frame 28 {
          }
          frame 29 {
          }
          frame 30 {
          }
          frame 31 {
          }
          frame 32 {
          }
          frame 33 {
          }
          frame 34 {
          }
          frame 37 {
          }
          frame 39 {
          }
          frame 40 {
          }
          frame 41 {
          }
          frame 42 {
          }
          frame 43 {
          }
          frame 50 {
          }
          frame 51 {
          }
          frame 52 {
          }
          frame 53 {
          }
          frame 54 {
          }
          frame 55 {
          }
          frame 56 {
          }
          frame 59 {
          }
          frame 65 {
          }
          frame 66 {
          }
          frame 67 {
          }
          frame 68 {
          }
          frame 69 {
          }
          frame 70 {
          }
          frame 73 {
          }
          frame 77 {
          }
          frame 78 {
          }
          frame 79 {
          }
        }
        n117 = Unbundle By Name(w577) -> ("status"=w586:bool)
        n118 = call "Run_Speed_Torque.vi"("Fault reset"=w585, "Network Path"=w557, "Torque Limit"=w587, "Speed Reference"=w582, "RUN REV."=w581, "RUN FOR."=w580) -> ("error out"=w589:errorcluster)  [unwired: 4 in, 1 out]
        n119 = call "Get Drive Status.vi"("Network Path"=w557) -> ("Fault"=w573:bool, "Alarm"=w572:bool, "error out"=w591:errorcluster)  [unwired: 1 in, 2 out]
        n120 = call "read model num.vi"("A1000 IP address"=w557) -> ("error out"=w592:errorcluster, "model string"=w584:string)  [unwired: 1 in]
        n121 = Unbundle By Name(w591) -> ("status"=w570:bool)
        n122 = Unbundle By Name(w592) -> ("status"=w571:bool)
        n123 = call <vilib>:"Clear Errors.vi"("error in (no error)"=w589, "specific error code to clear (0: all)"=0) -> ()  [unwired: 4 in, 2 out]
      }
      frame "500HP" {
        w714 = "192.168.1.22"  # Load IP Address
        # "Full scale HP"
        # "Full Scale Footpounds"
        # "Full Scale Rippums"
        n124 = call "Himmelstein_Read.vi"("connection ID"=w730, "error in (no error)"=w729) -> ("Torque"=w725:dbl, "Speed"=w727:dbl, "Power"=w726:dbl, "error out"=w728:errorcluster)  [unwired: 2 in, 1 out]
        n125 = Multiply(x=w734, y=10.0) -> (x*y=w736:dbl)
        n126 = Unbundle By Name(w728) -> ("status"=w743:bool)
        n127 = call "Run_Speed_Torque.vi"("Fault reset"=w735, "Network Path"=w714, "Torque Limit"=w736, "Speed Reference"=w732, "RUN REV."=w733, "RUN FOR."=w731) -> ("error out"=w738:errorcluster)  [unwired: 4 in, 1 out]
        n128 = call <vilib>:"EthernetIP CIP Get Attribute Single.vi"("Network Path"=w714, "Class"=125, "Instance"=u32 1, "Attribute"=128) -> ("Data"=w717:u8[], "error out"=w708:errorcluster)  [unwired: 9 in, 1 out]
        n129 = Unbundle By Name(w708) -> ("status"=w707:bool)
        n130 = Index Array(array=w717, index=0) -> (element=w715:u8)
        n131 = call <vilib>:"Clear Errors.vi"("error in (no error)"=w738, "specific error code to clear (0: all)"=0) -> ()  [unwired: 4 in, 2 out]
        n132 = case shown="56" w715 {
          tunnel: ["Unrecognized Fault" "--" "Uv1" "Uv2" "Uv3" "GF" "oC" "ov" "oH" "oH1" "oL1" "oL2" "oL3" "oL4" "rr" "rH" "EF3" "EF4" "EF5" "EF6" "EF7" "EF8" "oS" "dEv" "PGo" "PF" "LF" "oH3" "oPr" "Err" "oH4" "CE" "bUS" "CF" "EF0" "FbL" "UL3" "UL4" "oL7" "dv1" "dv2" "dv3" "dv4" "LF2" "STo" "PGoH" "SEr" "FbH" "EF1" "EF2" "oL5" "UL5" "CoF" "dwFL" "voF" "rF" "boL"] -> w713
          tunnel: ["Urecognized Fault" "No Fault Present" "DC Bus Undervolt" "CTL PS Undervolt" "MC Answerback" "Ground Fault" "Over Current" "DC Bus Overvolt" "Heatsink Overtemp" "Heatsink Max Temp" "Motor Overload" "Drive Overload" "Overtorque Det 1" "Overtorque Det 2" "DynBrk Transistor" "DynBrk Resistor" "External Fault 3" "External Fault 4" "External Fault 5" "External Fault 6" "External Fault 7" "External Fault 8" "Overspeed Det" "Speed Deviation" "PG Open" "Input Phase Loss" "Output Phase Loss" "Motor Overheat 1 (PTC Input)" "Operator Disconnected" "EEPROM R/W Error" "Motor OverHeat 2 (PTC Input)" "MEMOBUS/Modbus Com Fault" "EtherNet/IP Communication Error" "Out of Control" "External Fault 0" "PID Feedback Loss" "Undertorque Detection 1" "Undertorque Detection 2" "High Slip Braking oL" "Z Pulse Fault Detection" "Z pulse Noise Fault Detection" "Inversion Detection" "Inversion Prevention Detection" "Current Imbalance" "Pull-Out Detection" "PG Hardware Fault" "Too Many Speed Search Restarts" "Excessive PID Feedback" "External Fault (input terminal S1)" "External Fault (input terminal S2)" "Mechanical WeakeningDetection 1" "Mechanical Weakening Detection 2" "Current Offset Fault" "DriveWorksEZ Fault" "Output Voltage Detection Fault" "Braking Resistor Fault" "Braking Transistor Overload Fault"] -> _
          frame Default {
          }
          frame 0 {
          }
          frame 2 {
          }
          frame 3 {
          }
          frame 4 {
          }
          frame 6 {
          }
          frame 7 {
          }
          frame 8 {
          }
          frame 9 {
          }
          frame 10 {
          }
          frame 11 {
          }
          frame 12 {
          }
          frame 13 {
          }
          frame 14 {
          }
          frame 15 {
          }
          frame 16 {
          }
          frame 17 {
          }
          frame 18 {
          }
          frame 19 {
          }
          frame 20 {
          }
          frame 21 {
          }
          frame 22 {
          }
          frame 24 {
          }
          frame 25 {
          }
          frame 26 {
          }
          frame 27 {
          }
          frame 28 {
          }
          frame 29 {
          }
          frame 30 {
          }
          frame 31 {
          }
          frame 32 {
          }
          frame 33 {
          }
          frame 34 {
          }
          frame 37 {
          }
          frame 39 {
          }
          frame 40 {
          }
          frame 41 {
          }
          frame 42 {
          }
          frame 43 {
          }
          frame 50 {
          }
          frame 51 {
          }
          frame 52 {
          }
          frame 53 {
          }
          frame 54 {
          }
          frame 55 {
          }
          frame 56 {
          }
          frame 59 {
          }
          frame 65 {
          }
          frame 66 {
          }
          frame 67 {
          }
          frame 68 {
          }
          frame 69 {
          }
          frame 70 {
          }
          frame 73 {
          }
          frame 77 {
          }
          frame 78 {
          }
          frame 79 {
          }
        }
        n133 = call "Get Drive Status.vi"("Network Path"=w714) -> ("Fault"=w724:bool, "Alarm"=w723:bool, "error out"=w740:errorcluster)  [unwired: 1 in, 2 out]
        n134 = call "read model num.vi"("A1000 IP address"=w714) -> ("error out"=w741:errorcluster, "model string"=w742:string)  [unwired: 1 in]
        n135 = Unbundle By Name(w740) -> ("status"=w721:bool)
        n136 = Unbundle By Name(w741) -> ("status"=w722:bool)
      }
      frame "1200HP" {
        w859 = "192.168.1.23"  # Load IP Address
        # "Full scale HP"
        # "Full Scale Footpounds"
        # "Full Scale Rippums"
        n137 = call <vilib>:"EthernetIP CIP Get Attribute Single.vi"("Network Path"=w859, "Class"=125, "Instance"=u32 1, "Attribute"=128) -> ("Data"=w863:u8[], "error out"=w860:errorcluster)  [unwired: 9 in, 1 out]
        n138 = Unbundle By Name(w860) -> ()  [unwired: 1 out]
        n139 = Index Array(array=w863, index=0) -> (element=w861:u8)
        n140 = call "Himmelstein_Read.vi"("connection ID"=w881, "error in (no error)"=w880) -> ("Torque"=w876:dbl, "Speed"=w877:dbl, "Power"=w878:dbl, "error out"=w879:errorcluster)  [unwired: 2 in, 1 out]
        n141 = case shown="56" w861 {
          tunnel: ["Unrecognized Fault" "--" "Uv1" "Uv2" "Uv3" "GF" "oC" "ov" "oH" "oH1" "oL1" "oL2" "oL3" "oL4" "rr" "rH" "EF3" "EF4" "EF5" "EF6" "EF7" "EF8" "oS" "dEv" "PGo" "PF" "LF" "oH3" "oPr" "Err" "oH4" "CE" "bUS" "CF" "EF0" "FbL" "UL3" "UL4" "oL7" "dv1" "dv2" "dv3" "dv4" "LF2" "STo" "PGoH" "SEr" "FbH" "EF1" "EF2" "oL5" "UL5" "CoF" "dwFL" "voF" "rF" "boL"] -> w858
          tunnel: ["Urecognized Fault" "No Fault Present" "DC Bus Undervolt" "CTL PS Undervolt" "MC Answerback" "Ground Fault" "Over Current" "DC Bus Overvolt" "Heatsink Overtemp" "Heatsink Max Temp" "Motor Overload" "Drive Overload" "Overtorque Det 1" "Overtorque Det 2" "DynBrk Transistor" "DynBrk Resistor" "External Fault 3" "External Fault 4" "External Fault 5" "External Fault 6" "External Fault 7" "External Fault 8" "Overspeed Det" "Speed Deviation" "PG Open" "Input Phase Loss" "Output Phase Loss" "Motor Overheat 1 (PTC Input)" "Operator Disconnected" "EEPROM R/W Error" "Motor OverHeat 2 (PTC Input)" "MEMOBUS/Modbus Com Fault" "EtherNet/IP Communication Error" "Out of Control" "External Fault 0" "PID Feedback Loss" "Undertorque Detection 1" "Undertorque Detection 2" "High Slip Braking oL" "Z Pulse Fault Detection" "Z pulse Noise Fault Detection" "Inversion Detection" "Inversion Prevention Detection" "Current Imbalance" "Pull-Out Detection" "PG Hardware Fault" "Too Many Speed Search Restarts" "Excessive PID Feedback" "External Fault (input terminal S1)" "External Fault (input terminal S2)" "Mechanical WeakeningDetection 1" "Mechanical Weakening Detection 2" "Current Offset Fault" "DriveWorksEZ Fault" "Output Voltage Detection Fault" "Braking Resistor Fault" "Braking Transistor Overload Fault"] -> _
          frame Default {
          }
          frame 0 {
          }
          frame 2 {
          }
          frame 3 {
          }
          frame 4 {
          }
          frame 6 {
          }
          frame 7 {
          }
          frame 8 {
          }
          frame 9 {
          }
          frame 10 {
          }
          frame 11 {
          }
          frame 12 {
          }
          frame 13 {
          }
          frame 14 {
          }
          frame 15 {
          }
          frame 16 {
          }
          frame 17 {
          }
          frame 18 {
          }
          frame 19 {
          }
          frame 20 {
          }
          frame 21 {
          }
          frame 22 {
          }
          frame 24 {
          }
          frame 25 {
          }
          frame 26 {
          }
          frame 27 {
          }
          frame 28 {
          }
          frame 29 {
          }
          frame 30 {
          }
          frame 31 {
          }
          frame 32 {
          }
          frame 33 {
          }
          frame 34 {
          }
          frame 37 {
          }
          frame 39 {
          }
          frame 40 {
          }
          frame 41 {
          }
          frame 42 {
          }
          frame 43 {
          }
          frame 50 {
          }
          frame 51 {
          }
          frame 52 {
          }
          frame 53 {
          }
          frame 54 {
          }
          frame 55 {
          }
          frame 56 {
          }
          frame 59 {
          }
          frame 65 {
          }
          frame 66 {
          }
          frame 67 {
          }
          frame 68 {
          }
          frame 69 {
          }
          frame 70 {
          }
          frame 73 {
          }
          frame 77 {
          }
          frame 78 {
          }
          frame 79 {
          }
        }
        n142 = Unbundle By Name(w879) -> ("status"=w887:bool)
        n143 = Multiply(x=w883, y=10.0) -> (x*y=w889:dbl)
        n144 = call "Run_Speed_Torque.vi"("Fault reset"=w886, "Network Path"=w859, "Torque Limit"=w889, "Speed Reference"=w888, "RUN REV."=w884, "RUN FOR."=w882) -> ("error out"=w891:errorcluster)  [unwired: 4 in, 1 out]
        n145 = call "Get Drive Status.vi"("Network Path"=w859) -> ("Fault"=w875:bool, "Alarm"=w874:bool, "error out"=w893:errorcluster)  [unwired: 1 in, 2 out]
        n146 = call "read model num.vi"("A1000 IP address"=w859) -> ("error out"=w894:errorcluster, "model string"=w885:string)  [unwired: 1 in]
        n147 = Unbundle By Name(w893) -> ("status"=w872:bool)
        n148 = Unbundle By Name(w894) -> ("status"=w873:bool)
        n149 = call <vilib>:"Clear Errors.vi"("error in (no error)"=w891, "specific error code to clear (0: all)"=0) -> ()  [unwired: 4 in, 2 out]
      }
      frame "600HP" {
        w1010 = "192.168.1.23"  # Load IP Address
        # "Full scale HP"
        # "Full Scale Footpounds"
        # "Full Scale Rippums"
        n150 = call <vilib>:"EthernetIP CIP Get Attribute Single.vi"("Network Path"=w1010, "Class"=125, "Instance"=u32 1, "Attribute"=128) -> ("Data"=w1014:u8[], "error out"=w1011:errorcluster)  [unwired: 9 in, 1 out]
        n151 = Unbundle By Name(w1011) -> ()  [unwired: 1 out]
        n152 = Index Array(array=w1014, index=0) -> (element=w1012:u8)
        n153 = call "Himmelstein_Read.vi"("connection ID"=w1032, "error in (no error)"=w1031) -> ("Torque"=w1027:dbl, "Speed"=w1028:dbl, "Power"=w1029:dbl, "error out"=w1030:errorcluster)  [unwired: 2 in, 1 out]
        n154 = case shown="56" w1012 {
          tunnel: ["Unrecognized Fault" "--" "Uv1" "Uv2" "Uv3" "GF" "oC" "ov" "oH" "oH1" "oL1" "oL2" "oL3" "oL4" "rr" "rH" "EF3" "EF4" "EF5" "EF6" "EF7" "EF8" "oS" "dEv" "PGo" "PF" "LF" "oH3" "oPr" "Err" "oH4" "CE" "bUS" "CF" "EF0" "FbL" "UL3" "UL4" "oL7" "dv1" "dv2" "dv3" "dv4" "LF2" "STo" "PGoH" "SEr" "FbH" "EF1" "EF2" "oL5" "UL5" "CoF" "dwFL" "voF" "rF" "boL"] -> w1009
          tunnel: ["Urecognized Fault" "No Fault Present" "DC Bus Undervolt" "CTL PS Undervolt" "MC Answerback" "Ground Fault" "Over Current" "DC Bus Overvolt" "Heatsink Overtemp" "Heatsink Max Temp" "Motor Overload" "Drive Overload" "Overtorque Det 1" "Overtorque Det 2" "DynBrk Transistor" "DynBrk Resistor" "External Fault 3" "External Fault 4" "External Fault 5" "External Fault 6" "External Fault 7" "External Fault 8" "Overspeed Det" "Speed Deviation" "PG Open" "Input Phase Loss" "Output Phase Loss" "Motor Overheat 1 (PTC Input)" "Operator Disconnected" "EEPROM R/W Error" "Motor OverHeat 2 (PTC Input)" "MEMOBUS/Modbus Com Fault" "EtherNet/IP Communication Error" "Out of Control" "External Fault 0" "PID Feedback Loss" "Undertorque Detection 1" "Undertorque Detection 2" "High Slip Braking oL" "Z Pulse Fault Detection" "Z pulse Noise Fault Detection" "Inversion Detection" "Inversion Prevention Detection" "Current Imbalance" "Pull-Out Detection" "PG Hardware Fault" "Too Many Speed Search Restarts" "Excessive PID Feedback" "External Fault (input terminal S1)" "External Fault (input terminal S2)" "Mechanical WeakeningDetection 1" "Mechanical Weakening Detection 2" "Current Offset Fault" "DriveWorksEZ Fault" "Output Voltage Detection Fault" "Braking Resistor Fault" "Braking Transistor Overload Fault"] -> _
          frame Default {
          }
          frame 0 {
          }
          frame 2 {
          }
          frame 3 {
          }
          frame 4 {
          }
          frame 6 {
          }
          frame 7 {
          }
          frame 8 {
          }
          frame 9 {
          }
          frame 10 {
          }
          frame 11 {
          }
          frame 12 {
          }
          frame 13 {
          }
          frame 14 {
          }
          frame 15 {
          }
          frame 16 {
          }
          frame 17 {
          }
          frame 18 {
          }
          frame 19 {
          }
          frame 20 {
          }
          frame 21 {
          }
          frame 22 {
          }
          frame 24 {
          }
          frame 25 {
          }
          frame 26 {
          }
          frame 27 {
          }
          frame 28 {
          }
          frame 29 {
          }
          frame 30 {
          }
          frame 31 {
          }
          frame 32 {
          }
          frame 33 {
          }
          frame 34 {
          }
          frame 37 {
          }
          frame 39 {
          }
          frame 40 {
          }
          frame 41 {
          }
          frame 42 {
          }
          frame 43 {
          }
          frame 50 {
          }
          frame 51 {
          }
          frame 52 {
          }
          frame 53 {
          }
          frame 54 {
          }
          frame 55 {
          }
          frame 56 {
          }
          frame 59 {
          }
          frame 65 {
          }
          frame 66 {
          }
          frame 67 {
          }
          frame 68 {
          }
          frame 69 {
          }
          frame 70 {
          }
          frame 73 {
          }
          frame 77 {
          }
          frame 78 {
          }
          frame 79 {
          }
        }
        n155 = Unbundle By Name(w1030) -> ("status"=w1038:bool)
        n156 = Multiply(x=w1034, y=10.0) -> (x*y=w1040:dbl)
        n157 = call "Run_Speed_Torque.vi"("Fault reset"=w1037, "Network Path"=w1010, "Torque Limit"=w1040, "Speed Reference"=w1039, "RUN REV."=w1035, "RUN FOR."=w1033) -> ("error out"=w1042:errorcluster)  [unwired: 4 in, 1 out]
        n158 = call "Get Drive Status.vi"("Network Path"=w1010) -> ("Fault"=w1026:bool, "Alarm"=w1025:bool, "error out"=w1044:errorcluster)  [unwired: 1 in, 2 out]
        n159 = call "read model num.vi"("A1000 IP address"=w1010) -> ("error out"=w1045:errorcluster, "model string"=w1036:string)  [unwired: 1 in]
        n160 = Unbundle By Name(w1044) -> ("status"=w1023:bool)
        n161 = Unbundle By Name(w1045) -> ("status"=w1024:bool)
        n162 = call <vilib>:"Clear Errors.vi"("error in (no error)"=w1042, "specific error code to clear (0: all)"=0) -> ()  [unwired: 4 in, 2 out]
      }
    }
    "Load Drive:" <- w92
    "RPM" <- w65
    "LB-FT" <- w66
    "HP" <- w77
    n163 = Select(t=w7, s=w79, f=0.0) -> (s? t:f=→"% Torque":dbl)
    n164 = in-place {
      in-place-border: w59 -> [w212]
      in-place-border: w67 -> [w211]
      w219 = u32 0 ("Width")
      # "bar"
      n165 = Unbundle(T3 {"Width"=105, "Height"=105} ("cluster")) -> ("Width"=w215:u32, "Height"=w216:u32)
      n166 = Compound Arithmetic op=MULTIPLY(w212, invert w211, u16 360 ("value")) -> (w221:dbl)
      n167 = Bundle("Width"=w219, "Width"=w219, "Width"=w215, "Height"=w216) -> (w218:T4)  [unwired: 1 in]
      n168 = call <vilib>:"Draw Arc.vi"("rect"=w218) -> ("new picture"=w214:picture)  [unwired: 8 in]
      n169 = call <vilib>:"Draw Arc.vi"("picture"=w214, "start angle[degrees]"=i16 270, "rect"=w218, "fill?(F)"=TRUE, "color(black)"=u32 15204095, "arc size[degrees]"=w221) -> ("new picture"=→"2D Picture 7":picture)  [unwired: 3 in]
      "Numeric 10" <- w212
    }
    n170 = in-place {
      in-place-border: w17 -> [w226]
      # "fwd run"
      n171 = call <vilib>:"RGB to Color.vi"("B"=u8 80 ("R"), "G"=u8 72 ("R"), "R"=u8 47) -> ("Color"=w230:u32)
      n172 = call <vilib>:"RGB to Color.vi"("B"=u8 107 ("R"), "G"=u8 107 ("R"), "R"=u8 255) -> ("Color"=w234:u32)
      n173 = Select(t=w234, s=w226, f=w230) -> (s? t:f=w225:u32)
      n174 = property on="String 12" class="Str"("Text.TextColor"=w225) -> ()  [unwired: 2 in, 2 out]
    }
    n175 = in-place {
      in-place-border: w76 -> [w262]
      # "fwd run"
      n176 = call <vilib>:"RGB to Color.vi"("B"=u8 80 ("R"), "G"=u8 72 ("R"), "R"=u8 47) -> ("Color"=w266:u32)
      n177 = call <vilib>:"RGB to Color.vi"("B"=u8 107 ("R"), "G"=u8 107 ("R"), "R"=u8 255) -> ("Color"=w270:u32)
      n178 = Select(t=w270, s=w262, f=w266) -> (s? t:f=w261:u32)
      n179 = property on="String 10" class="Str"("Text.TextColor"=w261) -> ()  [unwired: 2 in, 2 out]
    }
    n180 = call "read parameters.vi"("A1000 IP address"=w90, "Select parameter"=T1."[E1-04] Maximum Output Frequency (V/f Pattern) [NUMERIC]") -> ("error out"=w88:errorcluster, "Current parameter setting"=w95:string)  [unwired: 4 in]
    n181 = call "read monitors_without U1-04.vi"("A1000 IP address"=w90, "Monitor Selection"=T2."output frequency [U1-02]") -> ("error out"=w89:errorcluster, "monitor string"=w93:string)  [unwired: 2 in]
    n182 = in-place {
      in-place-border: w66 -> [w286]
      in-place-border: w63 -> [w285]
      w293 = u32 0 ("Width")
      # "bar"
      n183 = Unbundle(T3 {"Width"=105, "Height"=105} ("cluster")) -> ("Width"=w289:u32, "Height"=w290:u32)
      n184 = Compound Arithmetic op=MULTIPLY(w286, invert w285, u16 360 ("value")) -> (w295:dbl)
      n185 = Bundle("Width"=w293, "Width"=w293, "Width"=w289, "Height"=w290) -> (w292:T4)  [unwired: 1 in]
      n186 = call <vilib>:"Draw Arc.vi"("rect"=w292) -> ("new picture"=w288:picture)  [unwired: 8 in]
      n187 = call <vilib>:"Draw Arc.vi"("picture"=w288, "start angle[degrees]"=i16 270, "rect"=w292, "fill?(F)"=TRUE, "color(black)"=u32 15204095, "arc size[degrees]"=w295) -> ("new picture"=→"2D Picture 5":picture)  [unwired: 3 in]
      "Numeric 8" <- w286
    }
    n188 = in-place {
      in-place-border: w77 -> [w272]
      in-place-border: w68 -> [w271]
      w279 = u32 0 ("Width")
      n189 = Unbundle(T3 {"Width"=105, "Height"=105} ("cluster")) -> ("Width"=w283:u32, "Height"=w282:u32)
      n190 = Compound Arithmetic op=MULTIPLY(w272, invert w271, u16 360 ("value")) -> (w277:dbl)
      n191 = Bundle("Width"=w279, "Width"=w279, "Width"=w283, "Height"=w282) -> (w280:T4)  [unwired: 1 in]
      n192 = call <vilib>:"Draw Arc.vi"("rect"=w280) -> ("new picture"=w284:picture)  [unwired: 8 in]
      n193 = call <vilib>:"Draw Arc.vi"("picture"=w284, "start angle[degrees]"=i16 270, "rect"=w280, "fill?(F)"=TRUE, "color(black)"=u32 15204095, "arc size[degrees]"=w277) -> ("new picture"=→"2D Picture 6":picture)  [unwired: 3 in]
      "Numeric 9" <- w272
    }
    n194 = in-place {
      in-place-border: w65 -> [w326]
      in-place-border: w64 -> [w325]
      w333 = u32 0 ("Width")
      n195 = Unbundle(T3 {"Width"=105, "Height"=105} ("cluster")) -> ("Width"=w337:u32, "Height"=w336:u32)
      n196 = Compound Arithmetic op=MULTIPLY(w326, invert w325, u16 360 ("value")) -> (w331:dbl)
      n197 = Bundle("Width"=w333, "Width"=w333, "Width"=w337, "Height"=w336) -> (w334:T4)  [unwired: 1 in]
      n198 = call <vilib>:"Draw Arc.vi"("rect"=w334) -> ("new picture"=w338:picture)  [unwired: 8 in]
      n199 = call <vilib>:"Draw Arc.vi"("picture"=w338, "start angle[degrees]"=i16 270, "rect"=w334, "fill?(F)"=TRUE, "color(black)"=u32 15204095, "arc size[degrees]"=w331) -> ("new picture"=→"2D Picture 4":picture)  [unwired: 3 in]
      "Numeric 7" <- w326
    }
    n200 = Fract/Exp String To Number(string=w95) -> ()  [unwired: 3 in, 2 out]
    n201 = Fract/Exp String To Number(string=w93) -> (number=w85:dbl)  [unwired: 3 in, 1 out]
    "Hz" <- w85
    n202 = Bundle(w85, 0.0) -> ()  [unwired: 1 in, 1 out]
    n203 = in-place {
      in-place-border: [w249] -> w99
      in-place-border: w98 -> [w248]
      in-place-border: w105 -> [w247]
      in-place-border: w69 -> [w246]
      n204 = property on="String 7" class="Str"("Text.Text"=w246) -> ()  [unwired: 2 in, 2 out]
      n205 = call <vilib>:"RGB to Color.vi"("B"=u8 80 ("R"), "G"=u8 73 ("R"), "R"=u8 47) -> ("Color"=w257:u32)
      n206 = call <vilib>:"RGB to Color.vi"("B"=u8 107 ("R"), "G"=u8 107 ("R"), "R"=u8 255) -> ("Color"=w253:u32)
      n207 = Select(t=w253, s=w247, f=w257) -> (s? t:f=w252:u32)
      n208 = Not(x=w248) -> (.not. x?=w249:bool)
      n209 = Select(t=w249, s=w247, f=TRUE) -> (s? t:f=w251:bool)
      n210 = property on="String 7" class="Str"("Text.Visible"=w251) -> ()  [unwired: 2 in, 2 out]
      n211 = property on="String 7" class="Str"("Text.TextColor"=w252) -> ()  [unwired: 2 in, 2 out]
    }
    n212 = Unbundle By Name(w89) -> ("status"=w31:bool)
    n213 = Unbundle By Name(w88) -> ("status"=w30:bool)
    n214 = Compound Arithmetic op=OR(w29, w28, w27, w31, w30) -> (w10:bool)
    n215 = And(x=w17, y=w11) -> (x .and. y?=w16:bool)
    n216 = And(x=w10, y=w11) -> (x .and. y?=w9:bool)
    n217 = in-place {
      in-place-border: w9 -> [w237]
      # "fwd run"
      n218 = property on="Network Error" class="Str"("Blinking"=FALSE) -> ()  [unwired: 2 in, 2 out]
      n219 = call <vilib>:"RGB to Color.vi"("B"=u8 80 ("R"), "G"=u8 72 ("R"), "R"=u8 47) -> ("Color"=w241:u32)
      n220 = call <vilib>:"RGB to Color.vi"("B"=u8 107 ("R"), "G"=u8 107 ("R"), "R"=u8 255) -> ("Color"=w245:u32)
      n221 = Select(t=w245, s=w237, f=w241) -> (s? t:f=w236:u32)
      n222 = property on="Network Error" class="Str"("Text.TextColor"=w236) -> ()  [unwired: 2 in, 2 out]
    }
    n223 = And(x=w19, y=w11) -> (x .and. y?=w18:bool)
    n224 = case shown="False" "OK Button" {
      tunnel: w18 -> [_ w123]
      tunnel: w16 -> [_ w122]
      tunnel: w9 -> [_ w121]
      frame False {
        w120 = FALSE ("Visible")
        n225 = property on="DAQ READ ERROR" class="Str"("Visible"=w120) -> ()  [unwired: 2 in, 2 out]
        n226 = property on="HIMMELSTEIN READ ERROR" class="Str"("Visible"=w120) -> ()  [unwired: 2 in, 2 out]
        n227 = property on="DRIVE READ ERROR" class="Str"("Visible"=w120) -> ()  [unwired: 2 in, 2 out]
      }
      frame True {
        n228 = case shown="True" w121 {
          frame False {
            n229 = property on="DRIVE READ ERROR" class="Str"("Visible"=FALSE) -> ()  [unwired: 2 in, 2 out]
          }
          frame True {
            n230 = property on="DRIVE READ ERROR" class="Str"("Visible"=TRUE) -> ()  [unwired: 2 in, 2 out]
          }
        }
        n231 = case shown="True" w122 {
          frame False {
            n232 = property on="HIMMELSTEIN READ ERROR" class="Str"("Visible"=FALSE) -> ()  [unwired: 2 in, 2 out]
          }
          frame True {
            n233 = property on="HIMMELSTEIN READ ERROR" class="Str"("Visible"=TRUE) -> ()  [unwired: 2 in, 2 out]
          }
        }
        n234 = case shown="True" w123 {
          frame False {
            n235 = property on="DAQ READ ERROR" class="Str"("Visible"=FALSE) -> ()  [unwired: 2 in, 2 out]
          }
          frame True {
            n236 = property on="DAQ READ ERROR" class="Str"("Visible"=TRUE) -> ()  [unwired: 2 in, 2 out]
          }
        }
      }
    }
    "DRIVE READ ERROR" <- "DRIVE READ ERRROR" ("DAQ READ ERROR")
    "HIMMELSTEIN READ ERROR" <- "HIMMELSTEIN READ ERRROR" ("DAQ READ ERROR")
    "DAQ READ ERROR" <- "DAQmx READ ERRROR" ("DAQ READ ERROR")
  }
